vi "GetControlValueHTTP.vi"(5 "num (false)":bool, 7 "Service":string="http://127.0.0.1/labview", 8 "error in":errorcluster, 10 "ctrl":string, 11 "vi":string) -> (0 "error out":errorcluster, 3 "value":string)   [LabVIEW 2021]
uses:
  <vilib>/httpClient/LabVIEWHTTPClient.lvlib
  <vilib>/wsapi/NI_WebServices.lvlib
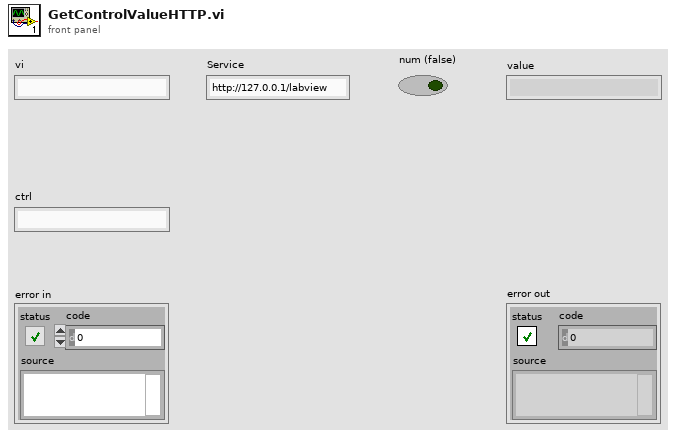
[diagram p1: front panel]
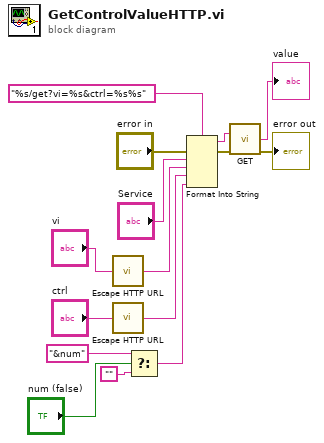
[diagram p0: block diagram]
diagram:
  n1 = call <vilib>:"Escape HTTP URL.vi"("unescaped string in"="vi") -> ("escaped string out"=w8:string)
  n2 = call <vilib>:"Escape HTTP URL.vi"("unescaped string in"="ctrl") -> ("escaped string out"=w6:string)
  n3 = Select(t="&num", s="num (false)", f="") -> (s? t:f=w10:string)
  n4 = Format Into String(format string="%s/get?vi=%s&ctrl=%s%s", error in="error in", "Service", w8, w6, w10) -> (resulting string=w5:string, error out=w2:errorcluster)  [unwired: 1 in]
  n5 = call <vilib>:"GET.vi"("url"=w5, "error in (no error)"=w2) -> ("body"=→"value":string, "error out"=→"error out":errorcluster)  [unwired: 10 in, 2 out]
